vi "ReadFreq.vi"(0 "reference in":refnum<class "Frequency_Counter_TTi.lvclass">, 5 "error in (no error)":errorcluster) -> (14 "reference in":refnum<class "Frequency_Counter_TTi.lvclass">, 16 "Frequency":dbl, 19 "error out":errorcluster)   [LabVIEW 2022 SP3, in "Frequency_Counter_TTi.lvlib" / "Frequency_Counter_TTi.lvclass"]
uses:
  Frequency_Counter_TTi.lvclass
  <vilib>/numeric/Random Number (Range) DBL.vi
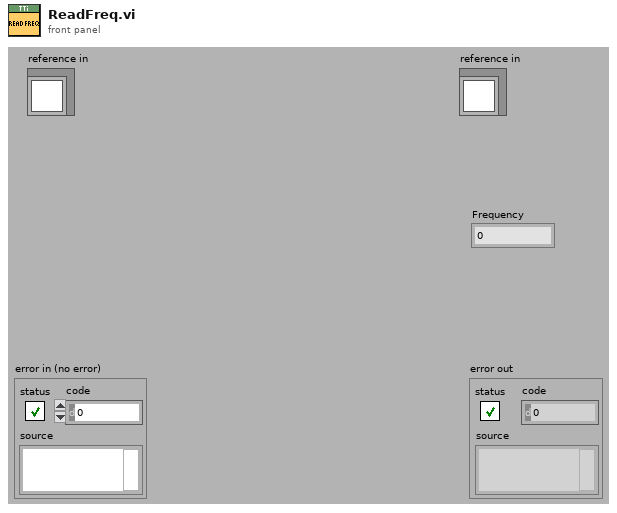
[diagram p1: front panel]
types:
  T1 = typedef "Frequency_Counter_TTi.lvlib/Frequency_Counter_TTi.lvclass/ObjectAttributes.ctl" = cluster{"Config":T2, "Freq":dbl}
  T2 = typedef "Frequency_Counter_TTi.lvlib/Frequency_Counter_TTi.lvclass/Config.ctl" = cluster{"ComPort":refnum<visa-resource-name>}
  T3 = typedef "Counter.lvlib/Counter.lvclass/ObjectAttributes.ctl" = cluster{"Config":T4, "Freq":dbl}
  T4 = typedef "Counter.lvlib/Counter.lvclass/Config.ctl" = cluster{"ComPort":refnum<visa-resource-name>}
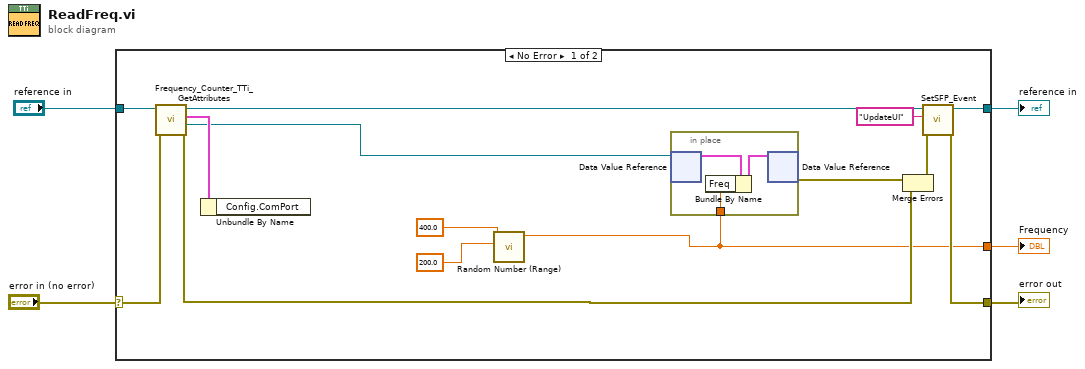
[diagram p0: block diagram]
diagram:
  n1 = case shown="No Error" "error in (no error)" {
    selector: "error in (no error)" -> [w19 w24]
    tunnel: [w13 w24] -> w4
    tunnel: [w14 w23] -> w2
    tunnel: "reference in" -> [w17 w23]
    tunnel: [w6 _] -> w1
    frame No Error {
      n2 = call "Frequency_Counter_TTi_GetAttributes.vi"("error in (no error)"=w19, "reference in"=w17) -> ("error out"=w7:errorcluster, "DataRef"=w16:refnum<data-value>, "Data"=w18:T1, "reference out"=w15:refnum<class "Frequency_Counter_TTi.lvclass">)  [unwired: 6 in]
      n3 = Unbundle By Name(w18) -> ()  [unwired: 1 out]
      n4 = call-poly <vilib>:"Random Number (Range).vi"("lower bound (0)"=200.0 ("frequency"), "upper bound (100)"=400.0 ("frequency")) -> ("number"=w6:dbl)  [unwired: 9 in]
      n5 = in-place {
        in-place-border: w6 -> [w20]
        n6 = in-place-dvr #1(w16) -> (w22:T3)  [unwired: 1 out]
        n7 = Bundle By Name(cluster=w22, "Freq"=w20) -> (w21:T3)
        n8 = in-place-dvr #1(w21) -> (w12:errorcluster)  [unwired: 1 out]
      }
      n9 = Merge Errors(w12, w7) -> (w11:errorcluster)
      n10 = call-dynamic "SetSFP_Event.vi"("error in (no error)"=w11, "msg"="UpdateUI", "reference in"=w15) -> ("error out"=w13:errorcluster, "reference out"=w14:refnum<class "Frequency_Counter_TTi.lvclass">)  [unwired: 7 in]
    }
    frame Error {
    }
  }
  "error out" <- w4
  "reference in" <- w2
  "Frequency" <- w1
